vi "Simulation Call Statechart.vi"(4 "operation":T1, 8 "error in":errorcluster, 10 "sensors":T3={"net distance (mm)"=0, "net angle (deg)"=0, "accelerometer"={"x axis (g)"=0.0, "y axis (g)"=0.0, "z axis (g)"=0.0}, "iRobot Sensors"={"Bumps + Wheel Drops"={"Wheeldrop Caster"=FALSE, "Wheeldrop Left"=FALSE, "Wheeldrop Right"=FALSE, "Bump Left"=FALSE, "Bump Right"=FALSE}, "Wall"=FALSE, "Cliff Left"=FALSE, "Cliff Front Left"=FALSE, "Cliff Front Right"=FALSE, "Cliff Right"=FALSE, "Wall Signal"=0, "Cliff Left Signal"=0, "Cliff Front Left Signal"=0, "Cliff Front Right Signal"=0, "Cliff Right Signal"=0, "Buttons"={"Advance"=FALSE, "Play"=FALSE}, "Virtual Wall"=FALSE, "# Stream Packets"=0, "Requested Velocity (mm/s)"=0, "Requested Radius (mm)"=0, "Requested Right Wheel Velocity (mm/s)"=0, "Requested Left Wheel Velocity (mm/s)"=0, "Distance (mm)"=0, "Angle (deg)"=0, "Song Playing"=FALSE, "Song Number"=0, "Charging State"=enum."Not Charging", "Voltage (mV)"=0, "Current (mA)"=0, "Battery Temperature (deg C)"=0, "Battery Charge (mAh)"=0, "Battery Capacity (mAh)"=0, "Charging Sources"={"Internal Charger"=FALSE, "Home Base"=FALSE}, "OI Mode"=enum."Off", "Digital Inputs"={"Digital Input 0"=FALSE, "Digital Input 1"=FALSE, "Digital Input 2"=FALSE, "Digital Input 3"=FALSE, "Device Detect"=FALSE}, "Drivers & Wheel Overcurrent"={"Low-Side Driver 0"=FALSE, "Low-Side Driver 1"=FALSE, "Low-Side Driver 2"=FALSE, "Left Wheel"=FALSE, "Right Wheel"=FALSE}, "Analog Signal"=0, "Infrared"=255}, "Is Simulator?"=FALSE} {"iRobot Sensors"."Infrared" format="%02x"; "accelerometer"."z axis (g)" format="%.3f"; "accelerometer"."y axis (g)" format="%.3f"; "accelerometer"."x axis (g)" format="%.3f"}, 11 "simulator":T15={"configuration"={"maxTime"=5.0, "enableVisualization"=TRUE, "statechart"=path "iRobot Navigation State Machine.vi", "environment"=path "iRobot Navigation State Machine.vi", "record"=path "Simulation Record.xml", "autograde?"=TRUE, "interactive?"=FALSE, "feedback mode"=enum."debug navigation"}, "Bump Sensors"=[], "Distance Sensors"=[], "Accelerometer"=refnum, "Wall Sensor"=refnum, "Statechart\ndisplay"=refnum, "Body"=refnum, "Left Motor"=refnum, "Right Motor"=refnum, "first step?"=FALSE}) -> (0 "error out":errorcluster, 2 "trace element":T2={"sensors"={"net distance (mm)"=0, "net angle (deg)"=0, "accelerometer"={"x axis (g)"=0.0, "y axis (g)"=0.0, "z axis (g)"=0.0}, "iRobot Sensors"={"Bumps + Wheel Drops"={"Wheeldrop Caster"=FALSE, "Wheeldrop Left"=FALSE, "Wheeldrop Right"=FALSE, "Bump Left"=FALSE, "Bump Right"=FALSE}, "Wall"=FALSE, "Cliff Left"=FALSE, "Cliff Front Left"=FALSE, "Cliff Front Right"=FALSE, "Cliff Right"=FALSE, "Wall Signal"=0, "Cliff Left Signal"=0, "Cliff Front Left Signal"=0, "Cliff Front Right Signal"=0, "Cliff Right Signal"=0, "Buttons"={"Advance"=FALSE, "Play"=FALSE}, "Virtual Wall"=FALSE, "# Stream Packets"=0, "Requested Velocity (mm/s)"=0, "Requested Radius (mm)"=0, "Requested Right Wheel Velocity (mm/s)"=0, "Requested Left Wheel Velocity (mm/s)"=0, "Distance (mm)"=0, "Angle (deg)"=0, "Song Playing"=FALSE, "Song Number"=0, "Charging State"=enum."Not Charging", "Voltage (mV)"=0, "Current (mA)"=0, "Battery Temperature (deg C)"=0, "Battery Charge (mAh)"=0, "Battery Capacity (mAh)"=0, "Charging Sources"={"Internal Charger"=FALSE, "Home Base"=FALSE}, "OI Mode"=enum."Off", "Digital Inputs"={"Digital Input 0"=FALSE, "Digital Input 1"=FALSE, "Digital Input 2"=FALSE, "Digital Input 3"=FALSE, "Device Detect"=FALSE}, "Drivers & Wheel Overcurrent"={"Low-Side Driver 0"=FALSE, "Low-Side Driver 1"=FALSE, "Low-Side Driver 2"=FALSE, "Left Wheel"=FALSE, "Right Wheel"=FALSE}, "Analog Signal"=0, "Infrared"=255}, "Is Simulator?"=FALSE}, "position"={"x (m)"=0.0, "y (m)"=0.0, "z (m)"=0.0}, "orientation"={"roll (deg)"=0.0, "pitch (deg)"=0.0, "yaw (deg)"=0.0}, "Simulation Time (s)"=0.0} {"sensors"."iRobot Sensors"."Infrared" format="%02x"; "sensors"."accelerometer"."z axis (g)" format="%.3f"; "sensors"."accelerometer"."y axis (g)" format="%.3f"; "sensors"."accelerometer"."x axis (g)" format="%.3f"}, 3 "simulator":T15={"configuration"={"maxTime"=5.0, "enableVisualization"=TRUE, "statechart"=path "iRobot Navigation State Machine.vi", "environment"=path "iRobot Navigation State Machine.vi", "record"=path "Simulation Record.xml", "autograde?"=TRUE, "interactive?"=FALSE, "feedback mode"=enum."debug navigation"}, "Bump Sensors"=[], "Distance Sensors"=[], "Accelerometer"=refnum, "Wall Sensor"=refnum, "Statechart\ndisplay"=refnum, "Body"=refnum, "Left Motor"=refnum, "Right Motor"=refnum, "first step?"=FALSE})   [LabVIEW 2013]
uses:
  shared/Sensors.ctl
  iRobot/Sensor/Accelerometer.ctl
  iRobot/Sensor/Sensor Group 6.ctl
  iRobot/Sensor/Bumps + Wheel Drops.ctl
  iRobot/Sensor/Buttons.ctl
  iRobot/Sensor/Charging State.ctl
  iRobot/Sensor/Charging Sources Available.ctl
  iRobot/Sensor/OI Mode.ctl
  iRobot/Sensor/Cargo Bay Digital Inputs.ctl
  iRobot/Sensor/Low-Side Driver + Wheel Overcurrent.ctl
  Simulator.ctl
  <instrlib>/DC Motor Controller/HAIOL/DC Motor Controller.lvclass
  CyberSim interface/Simulation Configuration.ctl
  autograder/feedbackMode.ctl
  Simulation Trace Element.ctl
  Simulated iRobot Position.ctl
  Simulated iRobot Orientation.ctl
  Simulation Call Statechart Operation.ctl
  Simulation Statechart Type.ctl
  Simulation Trace Operation.ctl
panel:
  # "Electrical: charging, battery, OI mode"
  # "Sensors: bump, cliff, button, wheel drop, wall, virtual wall"
  # "Motion: distance, angle, requested velocity"
  # "Cargo Bay: I/O, overcurrent, infrared"
  # "Song"
  # "Electrical: charging, battery, OI mode"
  # "Sensors: bump, cliff, button, wheel drop, wall, virtual wall"
  # "Motion: distance, angle, requested velocity"
  # "Cargo Bay: I/O, overcurrent, infrared"
  # "Song"
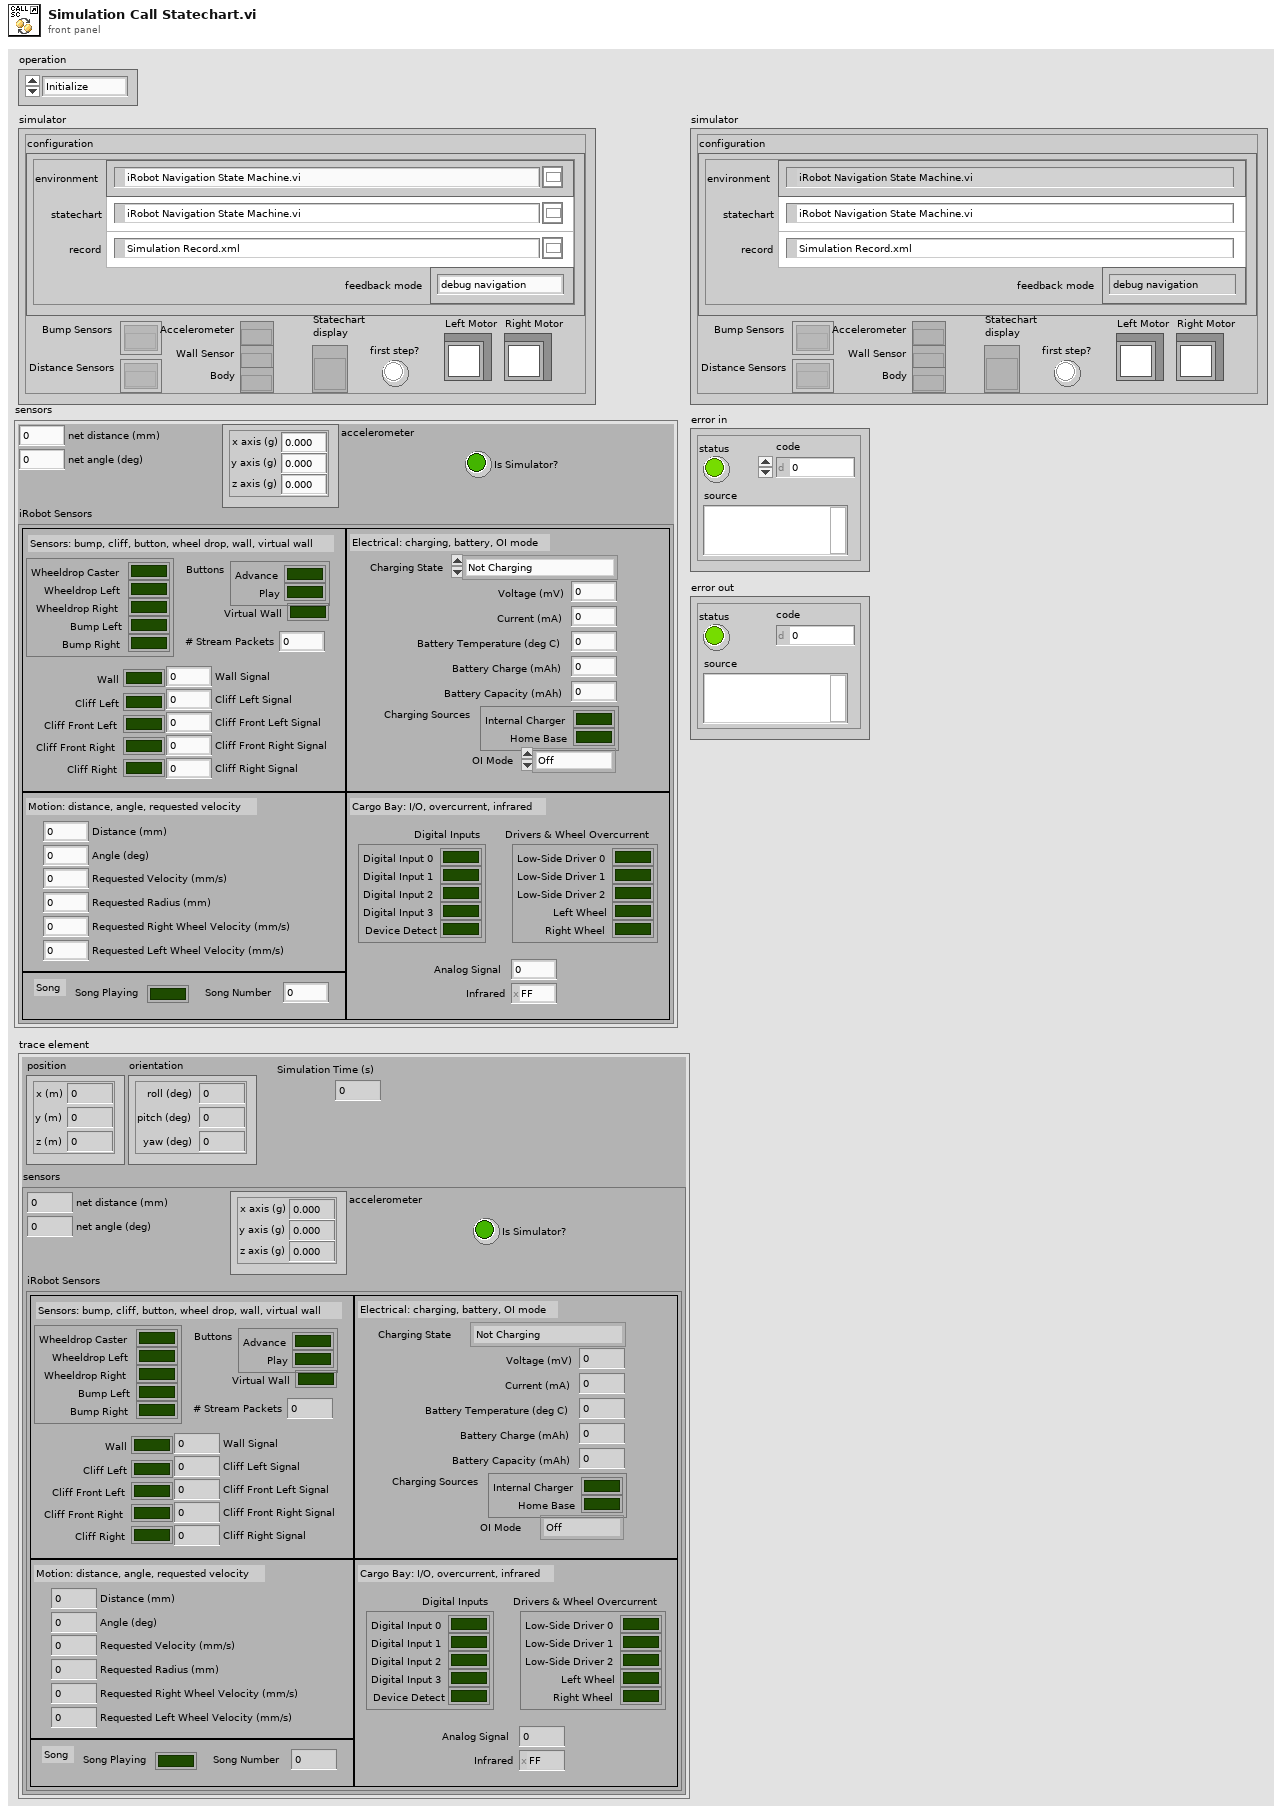
[diagram p1: front panel]
types:
  T1 = typedef "Simulation Call Statechart Operation.ctl" = enum16{"Initialize", "Call Statechart", "Finalize"}
  T2 = typedef "Simulation Trace Element.ctl" = cluster{"sensors":T3, "position":T13, "orientation":T14, "Simulation Time (s)":sgl}
  T3 = typedef "Sensors.ctl" = cluster{"net distance (mm)":i32, "net angle (deg)":i32, "accelerometer":T4, "iRobot Sensors":T5, "Is Simulator?":bool}
  T4 = typedef "Accelerometer.ctl" = cluster{"x axis (g)":dbl, "y axis (g)":dbl, "z axis (g)":dbl}
  T5 = typedef "Sensor Group 6.ctl" = cluster{"Bumps + Wheel Drops":T6, "Wall":bool, "Cliff Left":bool, "Cliff Front Left":bool, "Cliff Front Right":bool, "Cliff Right":bool, "Wall Signal":u16, "Cliff Left Signal":u16, "Cliff Front Left Signal":u16, "Cliff Front Right Signal":u16, "Cliff Right Signal":u16, "Buttons":T7, "Virtual Wall":bool, "# Stream Packets":u8, "Requested Velocity (mm/s)":i16, "Requested Radius (mm)":i16, "Requested Right Wheel Velocity (mm/s)":i16, "Requested Left Wheel Velocity (mm/s)":i16, "Distance (mm)":i32, "Angle (deg)":i32, "Song Playing":bool, "Song Number":u8, "Charging State":T8, "Voltage (mV)":u16, "Current (mA)":i16, "Battery Temperature (deg C)":i8, "Battery Charge (mAh)":u16, "Battery Capacity (mAh)":u16, "Charging Sources":T9, "OI Mode":T10, "Digital Inputs":T11, "Drivers & Wheel Overcurrent":T12, "Analog Signal":u16, "Infrared":u8}
  T6 = typedef "Bumps + Wheel Drops.ctl" = cluster{"Wheeldrop Caster":bool, "Wheeldrop Left":bool, "Wheeldrop Right":bool, "Bump Left":bool, "Bump Right":bool}
  T7 = typedef "Buttons.ctl" = cluster{"Advance":bool, "Play":bool}
  T8 = typedef "Charging State.ctl" = enum16{"Not Charging", "Reconditioning Charging", "Full Charging", "Trickle Charging", "Waiting", "Charging Fault Condition"}
  T9 = typedef "Charging Sources Available.ctl" = cluster{"Internal Charger":bool, "Home Base":bool}
  T10 = typedef "OI Mode.ctl" = enum16{"Off", "Passive", "Safe", "Full"}
  T11 = typedef "Cargo Bay Digital Inputs.ctl" = cluster{"Digital Input 0":bool, "Digital Input 1":bool, "Digital Input 2":bool, "Digital Input 3":bool, "Device Detect":bool}
  T12 = typedef "Low-Side Driver + Wheel Overcurrent.ctl" = cluster{"Low-Side Driver 0":bool, "Low-Side Driver 1":bool, "Low-Side Driver 2":bool, "Left Wheel":bool, "Right Wheel":bool}
  T13 = typedef "Simulated iRobot Position.ctl" = cluster{"x (m)":sgl, "y (m)":sgl, "z (m)":sgl}
  T14 = typedef "Simulated iRobot Orientation.ctl" = cluster{"roll (deg)":sgl, "pitch (deg)":sgl, "yaw (deg)":sgl}
  T15 = typedef "Simulator.ctl" = cluster{"configuration":T16, "Bump Sensors":refnum<k20>[], "Distance Sensors":refnum<k20>[], "Accelerometer":refnum<k20>, "Wall Sensor":refnum<k20>, "Statechart\ndisplay":refnum<vi>, "Body":refnum<k20>, "Left Motor":refnum<class "DC Motor Controller.lvclass">, "Right Motor":refnum<class "DC Motor Controller.lvclass">, "first step?":bool}
  T16 = typedef "Simulation Configuration.ctl" = cluster{"maxTime":sgl, "enableVisualization":bool, "statechart":path, "environment":path, "record":path, "autograde?":bool, "interactive?":bool, "feedback mode":T17}
  T17 = typedef "feedbackMode.ctl" = enum32{"debug navigation", "debug hill climb", "autograde navigation", "autograde hill climb"}
  T18 = typedef "Simulation Statechart Type.ctl" = enum16{"Unknown", "LabVIEW VI", "DLL"}
  T19 = typedef "Simulation Trace Operation.ctl" = enum16{"Initialize", "Record Trace Element", "Get Trace"}
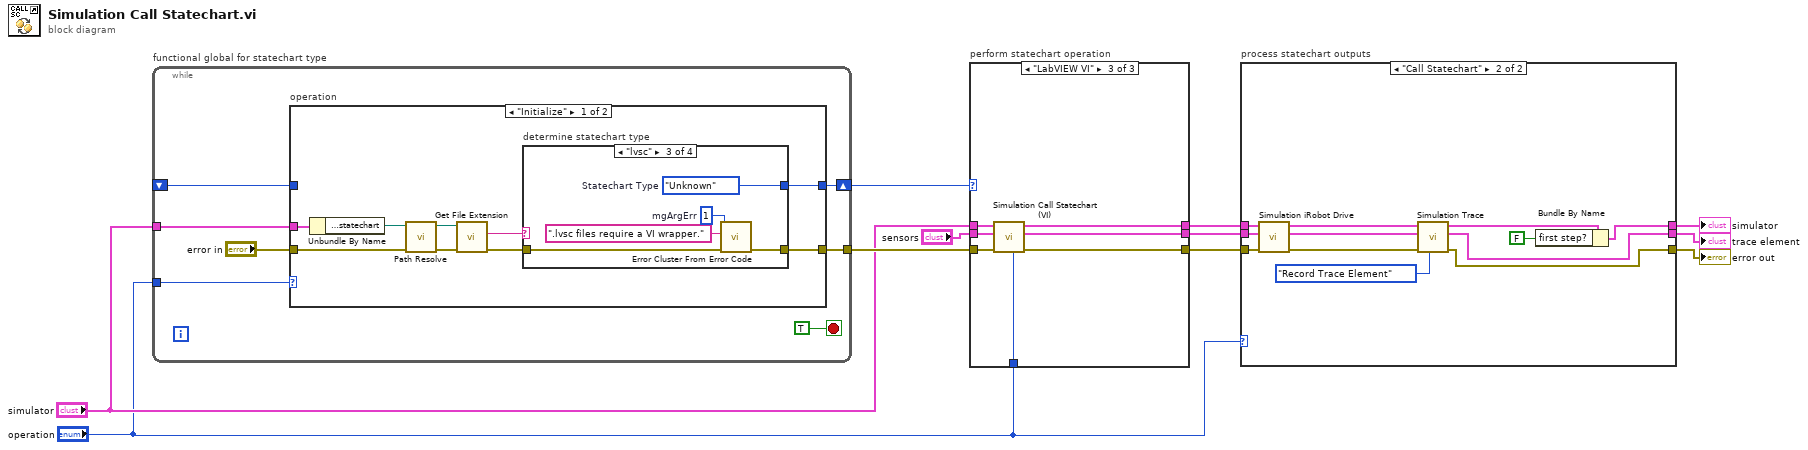
[diagram p0: block diagram]
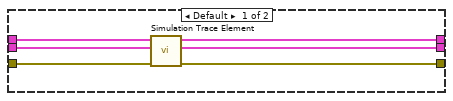
[diagram p2: hidden frame]
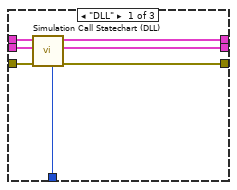
[diagram p3: hidden frame]
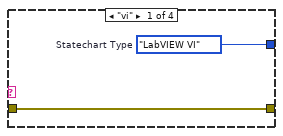
[diagram p5: hidden frame]
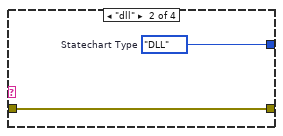
[diagram p6: hidden frame]
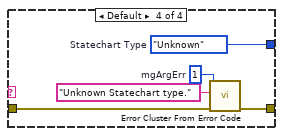
[diagram p7: hidden frame]
diagram:
  n1 = while "functional global for statechart type" {
    tunnel: "operation" -> [w12]
    tunnel: "simulator" -> [w18]
    shift-right: [w17] -> w11
    shift-left: _ -> [w15]
    tunnel: [w13] -> w10
    stop <- TRUE stop-if-true
    n2 = case "operation" shown="\"Initialize\"" w12 {
      tunnel: [w22 w43] -> w17
      tunnel: [w21 w42] -> w13
      tunnel: w18 -> [w20 _]
      tunnel: w15 -> [_ w43]
      tunnel: "error in" -> [w19 w42]
      frame "Initialize" {
        n3 = Unbundle By Name(w20) -> ("configuration.statechart"=w23:path)
        n4 = call "Path Resolve.vi"("Error In"=w19, "absolute or relative path"=w23) -> ("Error Out"=w25:errorcluster, "resolved path"=w24:path)  [unwired: 8 in]
        n5 = call <vilib>:"Get File Extension.vi"("error in (no error)"=w25, "file"=w24) -> ("error out"=w26:errorcluster, "lowercase file extension"=w27:string)  [unwired: 6 in, 2 out]
        n6 = case "determine statechart type" shown="\"lvsc\"" w27 {
          tunnel: w26 -> [w29 w31 w34 w39]
          tunnel: [w29 w31 w33 w38] -> w21
          tunnel: [w28 w30 w32 w37] -> w22
          frame "vi" {
            w28 = Simulation_Statechart_Type."LabVIEW VI"  # Statechart Type
          }
          frame "dll" {
            w30 = Simulation_Statechart_Type."DLL"  # Statechart Type
          }
          frame "lvsc" {
            w32 = Simulation_Statechart_Type."Unknown"  # Statechart Type
            w35 = 1  # mgArgErr
            n7 = call <vilib>:"Error Cluster From Error Code.vi"("error in (no error)"=w34, "error message (\"\")"=".lvsc files require a VI wrapper." ("error message (\"\")"), "error code (0)"=w35) -> ("error out"=w33:errorcluster)  [unwired: 6 in]
          }
          frame Default {
            w37 = Simulation_Statechart_Type."Unknown"  # Statechart Type
            w40 = 1  # mgArgErr
            n8 = call <vilib>:"Error Cluster From Error Code.vi"("error in (no error)"=w39, "error message (\"\")"="Unknown Statechart type." ("error message (\"\")"), "error code (0)"=w40) -> ("error out"=w38:errorcluster)  [unwired: 6 in]
          }
        }
      }
      frame Default {
      }
    }
  }
  n9 = case "perform statechart operation" shown="\"LabVIEW VI\"" w11 {
    tunnel: w10 -> [w48 w51 w58]
    tunnel: "simulator" -> [w50 w53 w60]
    tunnel: "operation" -> [w47 _ w54]
    tunnel: "sensors" -> [w49 w52 w59]
    tunnel: [w46 w53 w57] -> w6
    tunnel: [w45 w52 w56] -> w5
    tunnel: [w44 w51 w55] -> w4
    frame "DLL" {
      n10 = call "Simulation Call Statechart (DLL).vi"("operation"=w47, "error in (no error)"=w48, "sensors"=w49, "simulator"=w50) -> ("error out"=w44:errorcluster, "sensors"=w45:T3, "simulator"=w46:T15)  [unwired: 5 in]
    }
    frame "Unknown", Default {
    }
    frame "LabVIEW VI" {
      n11 = call "Simulation Call Statechart (VI).vi"("operation"=w54, "error in"=w58, "sensors"=w59, "simulator"=w60) -> ("error out"=w55:errorcluster, "sensors"=w56:T3, "simulator"=w57:T15)  [unwired: 5 in]
    }
  }
  n12 = case "process statechart outputs" shown="\"Call Statechart\"" "operation" {
    tunnel: w6 -> [w66 w72]
    tunnel: w5 -> [w62 w71]
    tunnel: w4 -> [w61 w70]
    tunnel: [w65 w69] -> w3
    tunnel: [w64 w68] -> w2
    tunnel: [w63 w67] -> w1
    frame Default {
      n13 = call "Simulation Trace Element.vi"("error in (no error)"=w61, "sensors"=w62, "simulator"=w66) -> ("error out"=w63:errorcluster, "trace element"=w64:T2, "simulator"=w65:T15)  [unwired: 6 in]
    }
    frame "Call Statechart" {
      n14 = call "Simulation iRobot Drive.vi"("error in"=w70, "sensors"=w71, "simulator in"=w72) -> ("error out"=w75:errorcluster, "sensors"=w76:T3, "simulator out"=w77:T15)  [unwired: 6 in]
      n15 = call "Simulation Trace.vi"("operation"=Simulation_Trace_Operation."Record Trace Element", "error in"=w75, "sensors"=w76, "simulator"=w77) -> ("error out"=w67:errorcluster, "last trace element"=w68:T2, "simulator"=w73:T15)  [unwired: 4 in, 1 out]
      n16 = Bundle By Name(cluster=w73, "first step?"=FALSE ("init?")) -> (w69:T15)
    }
  }
  "error out" <- w1
  "simulator" <- w3
  "trace element" <- w2
